vi "CodigoLabView 2_3.vi"() -> ()   [LabVIEW 2025]
uses:
  <vilib>/Utility/NIReport.llb/Report Type.ctl
  <vilib>/Instr/_visa.llb/VISA Configure Serial Port (Instr).vi
  <vilib>/addons/_office/excel.llb/Excel Easy Table (str).vi
  <vilib>/Utility/NIReport.llb/NI_report.lvclass
  <vilib>/Utility/NIReport.llb/NI_ReportGenerationCore.lvlib
  <vilib>/addons/_office/NI_ReportGenerationToolkit.lvlib
  <vilib>/Utility/NIReport.llb/Excel/NI_Excel.lvclass
panel:
  in  "template (empty)":path
  out "Tensión":string
  out "Rele 4":bool
  out "Estado 4":string
  out "Rele 3":bool
  out "Estado 3":string
  out "Rele 2":bool
  out "Estado 2":string
  out "rele 4":string
  in  "Relé N°4":bool
  out "rele 3":string
  in  "Relé N°3":bool
  out "rele 2":string
  in  "Relé N°2":bool
  out "Estado 1":string
  out "rele 1":string
  out "Rele 1":bool
  in  "Relé N°1":bool
  out "Serial Settings":u32
  out "error out 2":errorcluster
  out "Enviando":string
  out "error out":errorcluster
  in  "VISA resource name":refnum<visa-resource-name>
  in  "stop":bool
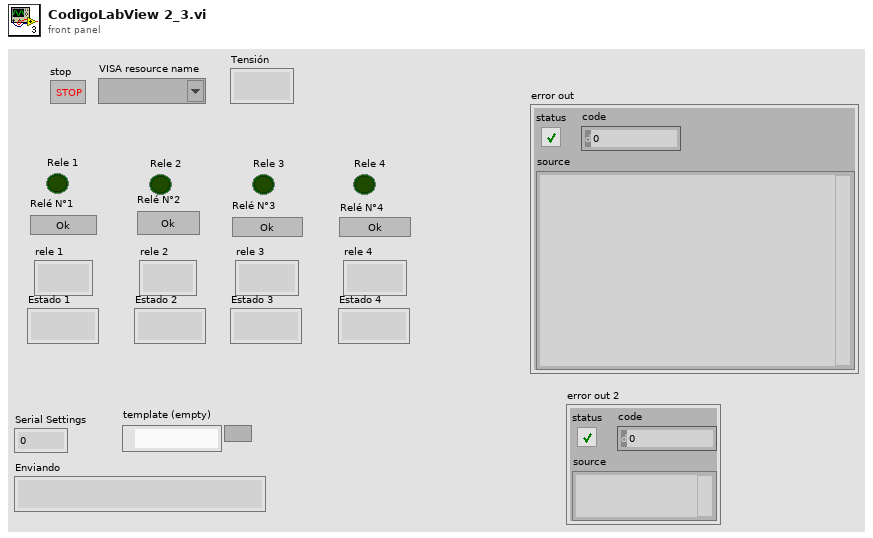
[diagram p1: front panel]
types:
  T1 = typedef "NI_ReportGenerationCore.lvlib/Report Type.ctl" = enum16{"HTML", "Word", "Excel"}
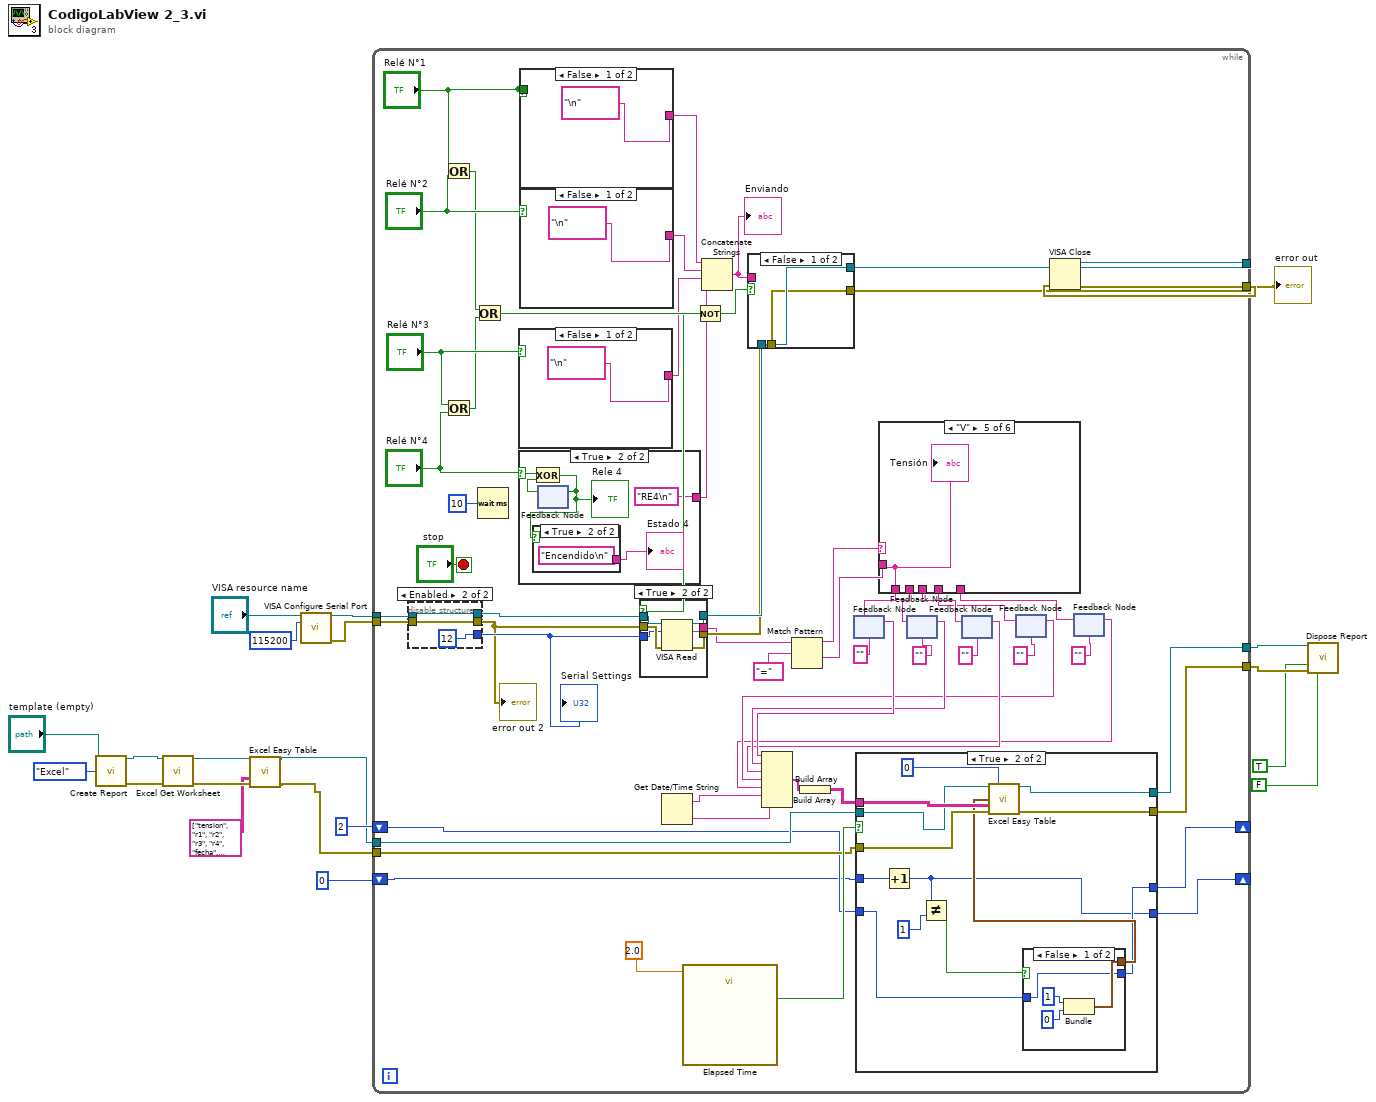
[diagram p0: block diagram]
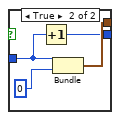
[diagram p3: hidden frame]
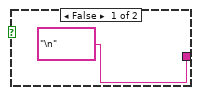
[diagram p4: hidden frame]
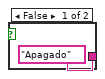
[diagram p5: hidden frame]
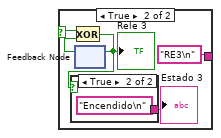
[diagram p6: hidden frame]
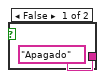
[diagram p7: hidden frame]
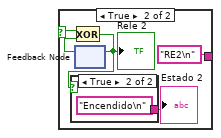
[diagram p8: hidden frame]
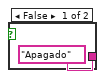
[diagram p9: hidden frame]
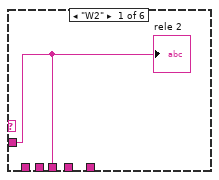
[diagram p10: hidden frame]
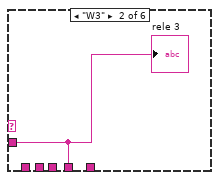
[diagram p11: hidden frame]
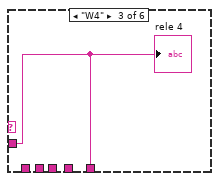
[diagram p12: hidden frame]
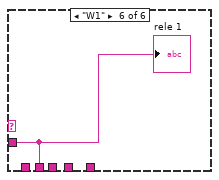
[diagram p14: hidden frame]
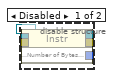
[diagram p15: hidden frame]
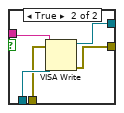
[diagram p17: hidden frame]
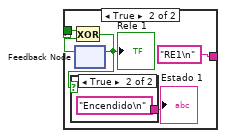
[diagram p18: hidden frame]
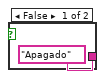
[diagram p19: hidden frame]
diagram:
  n1 = call <vilib>:"Create Report.vi"("report type"=Report_Type."Excel", "template (empty)"="template (empty)") -> ("report out"=w9:refnum<class "NI_report.lvclass">, "error out"=w8:errorcluster)  [unwired: 12 in]
  n2 = call <vilib>:"Excel Get Worksheet.vi"("report in"=w9, "error in (no error)"=w8) -> ("report out"=w3:refnum<class "NI_report.lvclass">, "error out"=w2:errorcluster)  [unwired: 12 in]
  n3 = call-poly <vilib>:"Excel Easy Table.vi"("report in"=w3, "text data"=string[][] [["tension", "r1", "r2", "r3", "r4", "fecha", "hora"]], "error in (no error)"=w2) -> ("report out"=w4:refnum<class "NI_report.lvclass">, "error out"=w5:errorcluster)  [unwired: 8 in, 3 out]
  n4 = call-poly "VISA Configure Serial Port"("VISA resource name"="VISA resource name", "baud rate (9600)"=u32 115200) -> ("VISA resource name out"=w22:refnum<visa-resource-name>, "error out"=w16:errorcluster)  [unwired: 12 in]
  n5 = while {
    tunnel: w22 -> [w78]
    tunnel: [w76] -> w21
    tunnel: w16 -> [w77]
    tunnel: [w75] -> w20
    tunnel: [w52] -> w13
    tunnel: [w51] -> w12
    tunnel: w4 -> [w45]
    tunnel: w5 -> [w44]
    shift-right: [w42] -> _
    shift-left: 2 -> [w43]
    shift-right: [w40] -> _
    shift-left: 0 -> [w41]
    stop <- "stop" stop-if-true
    n6 = disable-structure shown="Enabled" {
      disable-tunnel: w78 -> [w138 w141]
      disable-tunnel: w77 -> [w137 w140]
      disable-tunnel: [w136 w141] -> w72
      disable-tunnel: [w135 u32 12 ("Bytes at Port")] -> w71
      disable-tunnel: [w134 w140] -> w70
      frame Disabled {
        n7 = property class="Instr"(reference=w138, error in=w137) -> (reference out=w136:refnum<visa-resource-name>, error out=w134:errorcluster, "Serial Settings:Number of Bytes at Serial Port"=w135:u32)
      }
      frame Enabled {
      }
    }
    "error out 2" <- w70
    "Serial Settings" <- w71
    n8 = Or(x="Relé N°1", y="Relé N°2") -> (x .or. y?=w61:bool)
    n9 = Or(x="Relé N°3", y="Relé N°4") -> (x .or. y?=w60:bool)
    n10 = Or(x=w61, y=w60) -> (x .or. y?=w65:bool)
    n11 = Wait (ms)(milliseconds to wait=u32 10) -> ()  [unwired: 1 out]
    n12 = case shown="False" "Relé N°3" {
      selector: "Relé N°3" -> [_ w114]
      tunnel: ["\n" "RE3\n"] -> w59
      frame False {
      }
      frame True {
        n13 = feedback #1() -> (w117:bool)  [unwired: 1 in]
        n14 = Exclusive Or(1:w117, 2:w114) -> (0:w116:bool)
        "Rele 3" <- w116
        n15 = case shown="True" w116 {
          tunnel: ["Apagado" "Encendido\n"] -> w115
          frame False {
          }
          frame True {
          }
        }
        "Estado 3" <- w115
        n16 = feedback-in #1(w116) -> ()
      }
    }
    n17 = case shown="True" "Relé N°4" {
      selector: "Relé N°4" -> [_ w106]
      tunnel: ["\n" "RE4\n"] -> w58
      frame False {
      }
      frame True {
        n18 = feedback #2() -> (w109:bool)  [unwired: 1 in]
        n19 = Exclusive Or(1:w109, 2:w106) -> (0:w108:bool)
        "Rele 4" <- w108
        n20 = case shown="True" w108 {
          tunnel: ["Apagado" "Encendido\n"] -> w107
          frame False {
          }
          frame True {
          }
        }
        "Estado 4" <- w107
        n21 = feedback-in #2(w108) -> ()
      }
    }
    n22 = case shown="False" "Relé N°1" {
      tunnel: ["\n" "RE1\n"] -> w56
      tunnel: "Relé N°1" -> [_ w161]
      frame False {
      }
      frame True {
        n23 = feedback #3() -> (w160:bool)  [unwired: 1 in]
        n24 = Exclusive Or(1:w160, 2:w161) -> (0:w159:bool)
        "Rele 1" <- w159
        n25 = case shown="True" w159 {
          tunnel: ["Apagado" "Encendido\n"] -> w158
          frame False {
          }
          frame True {
          }
        }
        "Estado 1" <- w158
        n26 = feedback-in #3(w159) -> ()
      }
    }
    n27 = case shown="False" "Relé N°2" {
      selector: "Relé N°2" -> [_ w122]
      tunnel: ["\n" "RE2\n"] -> w57
      frame False {
      }
      frame True {
        n28 = feedback #4() -> (w125:bool)  [unwired: 1 in]
        n29 = Exclusive Or(1:w125, 2:w122) -> (0:w124:bool)
        "Rele 2" <- w124
        n30 = case shown="True" w124 {
          tunnel: ["Apagado" "Encendido\n"] -> w123
          frame False {
          }
          frame True {
          }
        }
        "Estado 2" <- w123
        n31 = feedback-in #4(w124) -> ()
      }
    }
    n32 = Get Date/Time String() -> (date string=w47:string, time string=w46:string)  [unwired: 3 in]
    n33 = call "Elapsed Time"("Time Target (s)"=2.0) -> ("Time has Elapsed"=w48:bool)  [unwired: 11 in, 7 out]
    n34 = Not(x=w65) -> (.not. x?=w50:bool)
    n35 = case shown="True" w50 {
      tunnel: [w143 w149] -> w74
      tunnel: [w142 w148] -> w73
      tunnel: w70 -> [w142 w147]
      tunnel: w72 -> [w143 w146]
      tunnel: w71 -> [_ w145]
      tunnel: [_ w144] -> w39
      frame False {
      }
      frame True {
        n36 = VISA Read(VISA resource name=w146, byte count=w145, error in (no error)=w147) -> (VISA resource name out=w149:refnum<visa-resource-name>, read buffer=w144:string, error out=w148:errorcluster)  [unwired: 1 out]
      }
    }
    n37 = Concatenate Strings(w56, w57, w59, w58) -> (w55:string)
    "Enviando" <- w55
    n38 = case shown="False" w65 {
      tunnel: [w151 w156] -> w76
      tunnel: [w150 w155] -> w75
      tunnel: w74 -> [w151 w154]
      tunnel: w73 -> [w150 w153]
      tunnel: w55 -> [_ w152]
      frame False {
      }
      frame True {
        n39 = VISA Write(VISA resource name=w154, write buffer=w152, error in (no error)=w153) -> (VISA resource name out=w156:refnum<visa-resource-name>, error out=w155:errorcluster)  [unwired: 1 out]
      }
    }
    n40 = Match Pattern(string=w39, regular expression="=") -> (before substring=w67:string, after substring=w38:string)  [unwired: 1 in, 2 out]
    n41 = feedback #5("" ("read buffer")) -> (w37:string)
    n42 = case shown="\"V\"" w67 {
      tunnel: w38 -> [w129 w130 w131 _ w132 w133]
      tunnel: [_ _ _ _ w132 _] -> w35
      tunnel: [_ _ _ _ _ w133] -> w34
      tunnel: [w129 _ _ _ _ _] -> w32
      tunnel: [_ w130 _ _ _ _] -> w30
      tunnel: [_ _ w131 _ _ _] -> w28
      frame "W2" {
        "rele 2" <- w129
      }
      frame "W3" {
        "rele 3" <- w130
      }
      frame "W4" {
        "rele 4" <- w131
      }
      frame "False", Default {
      }
      frame "V" {
        "Tensión" <- w132
      }
      frame "W1" {
        "rele 1" <- w133
      }
    }
    n43 = feedback-in #5(w35) -> ()
    n44 = feedback #6("" ("read buffer")) -> (w33:string)
    n45 = feedback-in #6(w34) -> ()
    n46 = feedback #7("" ("read buffer")) -> (w31:string)
    n47 = feedback-in #7(w32) -> ()
    n48 = feedback #8("" ("read buffer")) -> (w29:string)
    n49 = feedback-in #8(w30) -> ()
    n50 = feedback #9("" ("read buffer")) -> (w27:string)
    n51 = Build Array(w37, w33, w31, w29, w27, w47, w46) -> (w54:string[])
    n52 = Build Array(w54) -> (w53:string[][])
    n53 = case shown="True" w48 {
      tunnel: w53 -> [_ w96]
      tunnel: w44 -> [w83 w95]
      tunnel: [w82 w94] -> w52
      tunnel: [w83 w93] -> w51
      tunnel: w45 -> [w82 w92]
      tunnel: w43 -> [w81 w89]
      tunnel: [w81 w88] -> w42
      tunnel: w41 -> [w80 w87]
      tunnel: [w80 w84] -> w40
      frame False {
      }
      frame True {
        n54 = Increment(x=w87) -> (x+1=w84:i32)
        n55 = Not Equal?(x=w84, y=1) -> (x != y?=w85:bool)
        n56 = case shown="False" w85 {
          tunnel: [w98 w104] -> w91
          tunnel: w89 -> [w97 w102]
          tunnel: [w97 w101] -> w88
          frame False {
            n57 = Bundle(1, 0) -> (w98:cluster{i32, i32})  [unwired: 1 in]
          }
          frame True {
            n58 = Increment(x=w102) -> (x+1=w101:i32)
            n59 = Bundle(w102, 0) -> (w104:cluster{i32, i32})  [unwired: 1 in]
          }
        }
        n60 = call-poly <vilib>:"Excel Easy Table.vi"("report in"=w92, "iteration"=0, "start (0, 0)"=w91, "text data"=w96, "error in (no error)"=w95) -> ("report out"=w94:refnum<class "NI_report.lvclass">, "error out"=w93:errorcluster)  [unwired: 6 in, 3 out]
      }
    }
    n61 = feedback-in #9(w28) -> ()
  }
  n62 = VISA Close(VISA resource name=w21, error in (no error)=w20) -> (error out=→"error out":errorcluster)
  n63 = call-dynamic "Dispose Report.vi"("report in"=w13, "save changes? (F)"=TRUE, "error in (no error)"=w12, "close report? (T)"=FALSE) -> ()  [unwired: 11 in, 1 out]
